vi "initilize.vi"(8 "error in (no error)":errorcluster, 9 "Serial device Brand":T1, 10 "VISA resource name":refnum<visa-resource-name>, 11 "Arduino in":refnum<class "Arduino.lvclass">) -> (0 "error out":errorcluster, 3 "Arduino out":refnum<class "Arduino.lvclass">)   [LabVIEW 2019, in "Arduino.lvclass"]
uses:
  Arduino.lvclass
  Control 14.ctl
  Arduino.lvclass/Arduino.ctl
  <vilib>/Instr/_visa.llb/VISA Configure Serial Port (Instr).vi
  Serial Device.lvclass
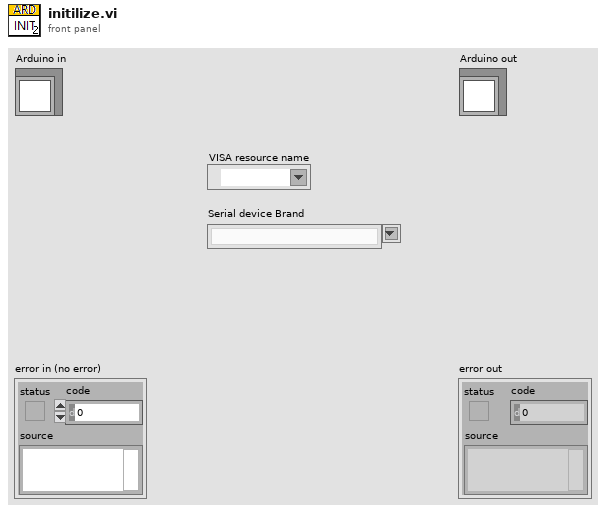
[diagram p1: front panel]
types:
  T1 = typedef "Serial Device.lvclass/Control 14.ctl" = string
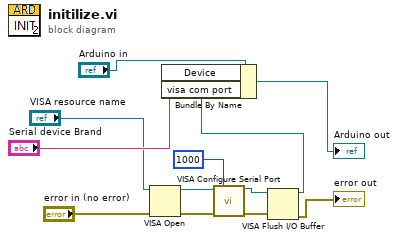
[diagram p0: block diagram]
diagram:
  n1 = VISA Open(error in (no error)="error in (no error)", VISA resource name="VISA resource name") -> (VISA resource name=w8:refnum<visa-resource-name>, error out=w3:errorcluster)  [unwired: 3 in]
  n2 = call-poly "VISA Configure Serial Port"("VISA resource name"=w8, "timeout (10sec)"=u32 1000, "error in (no error)"=w3) -> ("VISA resource name out"=w5:refnum<visa-resource-name>, "error out"=w2:errorcluster)  [unwired: 11 in]
  n3 = VISA Flush I/O Buffer(VISA resource name=w5, error in (no error)=w2) -> (VISA resource name out=w4:refnum<visa-resource-name>, error out=→"error out":errorcluster)  [unwired: 1 in]
  n4 = Bundle By Name(cluster="Arduino in", "Device"="Serial device Brand", "visa com port"=w4) -> (→"Arduino out":refnum<class "Arduino.lvclass">)
